vi "GetBars.vi"(8 "error in (no error)":errorcluster, 10 "Munged Input":string, 11 "Code39 in":refnum<class "Code39.lvclass">) -> (0 "error out":errorcluster, 2 "Bars":T1[][](array[typedef]), 3 "Code39 out":refnum<class "Code39.lvclass">)   [LabVIEW 2013, in "BarCodes.lvlib" / "Code39.lvclass"]
doc: "Gets the bars of the bar code. The bars are specified as an array of bar widths from left to right."
uses:
  Code39.lvclass
  BarCode/Bar.ctl
  Code39.lvclass/Code39.ctl
  BarCode/BarCode.lvclass
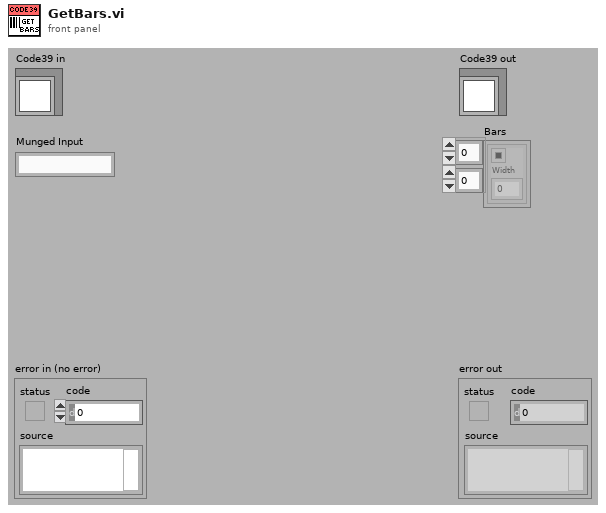
[diagram p1: front panel]
types:
  T1 = typedef "BarCodes.lvlib/BarCode.lvclass/Bar.ctl" = cluster{"Color":u32, "Width":u8}
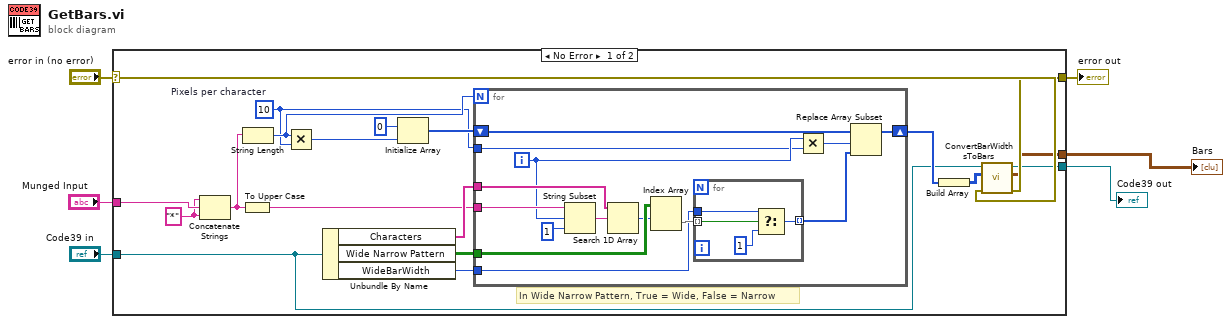
[diagram p0: block diagram]
diagram:
  n1 = case shown="No Error" "error in (no error)" {
    selector: "error in (no error)" -> [w10 w45]
    tunnel: "Code39 in" -> [w11 w44]
    tunnel: "Munged Input" -> [w17 _]
    tunnel: [w9 w45] -> w3
    tunnel: [w8 w44] -> w2
    tunnel: [w7 _] -> w1
    frame No Error {
      w16 = "*" ("string")
      w14 = 10  # Pixels per character
      # "In Wide Narrow Pattern, True = Wide, False = Narrow"
      n2 = Concatenate Strings(w16, w17, w16) -> (w15:string)
      n3 = To Upper Case(1:w15) -> (0:w19:string)
      n4 = String Length(string=w15) -> (length=w23:i32)
      n5 = Multiply(x=w23, y=w14) -> (x*y=w21:i32)
      n6 = Unbundle By Name(w11) -> ("Characters"=w25:string[], "Wide Narrow Pattern"=w24:bool[][], "WideBarWidth"=w18:u8)
      n7 = Initialize Array(u8 0 ("Numeric"), w21) -> (w20:u8[])
      n8 = for {
        N: w23 -> [_]
        tunnel: w19 -> [w39]
        tunnel: w25 -> [w37]
        tunnel: w24 -> [w35]
        shift-right: [w28] -> w12
        shift-left: w20 -> [w33]
        tunnel: w18 -> [w27]
        tunnel: w14 -> [w26]
        i -> [w32]
        n9 = String Subset(string=w39, offset (0)=w32, length (rest)=1 ("length (rest)")) -> (substring=w36:string)
        n10 = Search 1D Array(1D array=w37, element=w36) -> (index of element=w34:i32)  [unwired: 1 in]
        n11 = Index Array(array=w35, index (row)=w34) -> (element=w30:bool[])  [unwired: 1 in]
        n12 = for {
          tunnel: w30 -> [w43] mode=indexing
          tunnel: [w41] -> w29 mode=indexing
          tunnel: w27 -> [w40]
          n13 = Select(t=w40, s=w43, f=u8 1 ("Numeric")) -> (s? t:f=w41:u8)
        }
        n14 = Multiply(x=w32, y=w26) -> (x*y=w31:i32)
        n15 = Replace Array Subset(array=w33, new element=w29, index=w31) -> (w28:u8[])
      }
      n16 = Build Array(w12) -> (w13:u8[][])
      n17 = call "ConvertBarWidthsToBars.vi"("error in (no error)"=w10, "BarWidths"=w13, "BarCode in"=w11) -> ("error out"=w9:errorcluster, "Bars"=w7:T1[][], "BarCode out"=w8:refnum<class "Code39.lvclass">)  [unwired: 6 in]
    }
    frame Error {
    }
  }
  "error out" <- w3
  "Code39 out" <- w2
  "Bars" <- w1
